vi "Read Configuration Parameter.vi"(8 "error in (no error)":errorcluster, 11 "RandomNumberGenerator in":refnum<class "RandomNumberGenerator.lvclass">) -> (0 "error out":errorcluster, 2 "Configuration":T1, 3 "RandomNumberGenerator out":refnum<class "RandomNumberGenerator.lvclass">)   [LabVIEW 2020, in "RandomNumberGenerator.lvlib" / "RandomNumberGenerator.lvclass"]
doc: "<b>Read Configuration Parameter</b>\nThis method returns the configuration parameter from the class data for this plugin. It is returned as a populated <b>Configuration.ctl</b> from this plugin."
uses:
  RandomNumberGenerator.lvclass
  C:/Program Files/National Instruments/LabVIEW 2020/vi.lib/FlexLogger/SDK/PluginSDK.lvlibp/PEFClasses/SDK/Processing Element/Processing Element.lvclass
  Configuration.ctl
  Get Configuration Version.vi
  Mutate Configuration to Current.vi
  Default Configuration Parameters.vi
  <vilib>/FlexLogger/SDK/PluginSDK.lvlibp/PEFClasses/SDK/Processing Element/Read Parameters Property.vi
  <vilib>/FlexLogger/SDK/PluginSDK.lvlibp/PEFClasses/SDK/Parameters/PolyHelpers/GetParameter(String).vi
  <vilib>/ADAS Record/Utilities/Config/Data Converter/Populate Container from JSON.vi
  <vilib>/FlexLogger/SDK/PluginSDK.lvlibp/PEFClasses/SDK/Parameters/Parameters.lvclass
panel:
  # "#via_ignore"
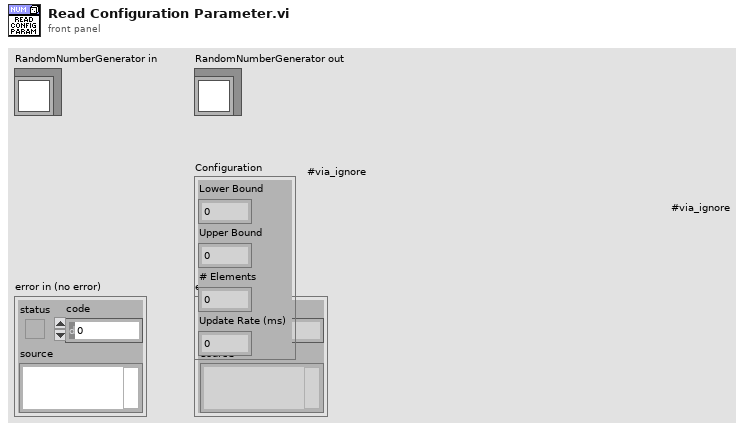
[diagram p1: front panel]
types:
  T1 = typedef "RandomNumberGenerator.lvlib/RandomNumberGenerator.lvclass/Configuration.ctl" = cluster{"Lower Bound":dbl, "Upper Bound":dbl, "# Elements":i32, "Update Rate (ms)":i32}
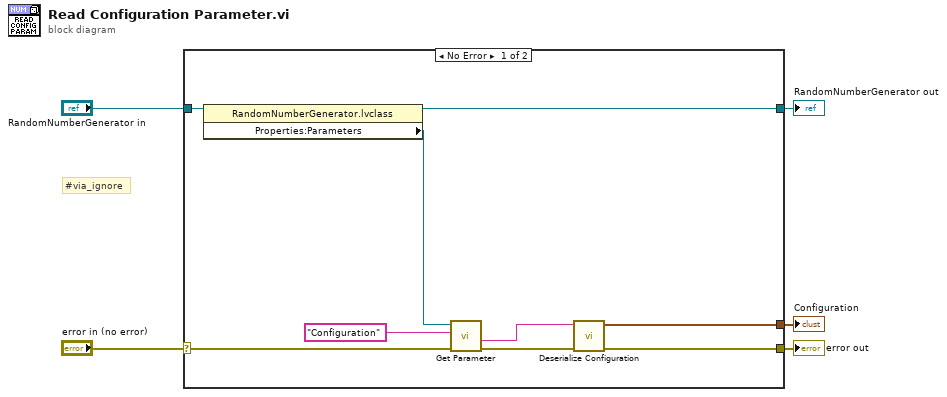
[diagram p0: block diagram]
diagram:
  # "#via_ignore"
  n1 = case shown="No Error" "error in (no error)" {
    selector: "error in (no error)" -> [w8 w16]
    tunnel: [w7 w16] -> w4
    tunnel: [w9 w15] -> w2
    tunnel: "RandomNumberGenerator in" -> [w10 w15]
    tunnel: [w6 _] -> w1
    frame No Error {
      n2 = property on="Property Node" class="RandomNumberGenerator.lvclass"(reference=w10) -> (reference out=w9:refnum<class "RandomNumberGenerator.lvclass">, "Properties:Parameters"=w14:refnum<class "Parameters.lvclass">)  [unwired: 1 in, 1 out]
      n3 = call-poly <vilib>:"Get Parameter.vi"("error in (no error)"=w8, "Name"="Configuration", "Parameters in"=w14) -> ("error out"=w12:errorcluster, "Value"=w11:string)  [unwired: 5 in, 2 out]
      n4 = call "Deserialize Configuration.vi"("error in (no error)"=w12, "Serialized Configuration"=w11) -> ("error out"=w7:errorcluster, "Configuration"=w6:T1)  [unwired: 8 in]
    }
    frame Error {
    }
  }
  "error out" <- w4
  "RandomNumberGenerator out" <- w2
  "Configuration" <- w1
